vi "Test_uart.vi"() -> ()   [LabVIEW 2025]
uses:
  <vilib>/Instr/_visa.llb/VISA Configure Serial Port (Instr).vi
panel:
  in  "Stop Button":bool
  out "Waveform Chart":cluster{"Número":sgl, "Número":sgl}(graph)
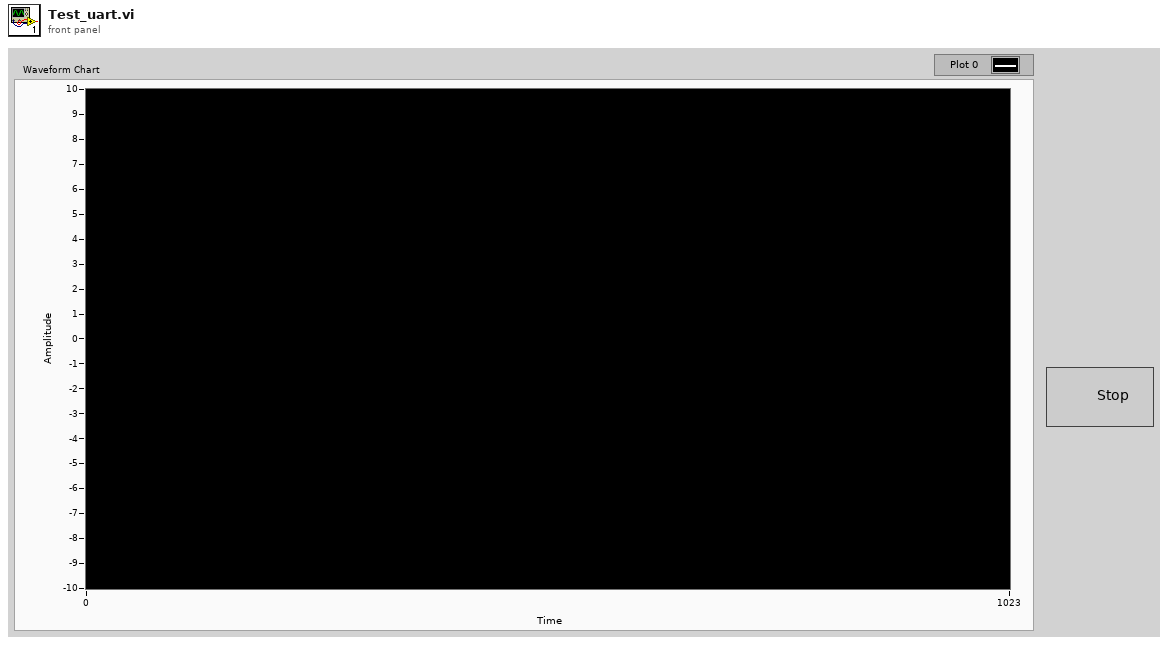
[diagram p1: front panel]
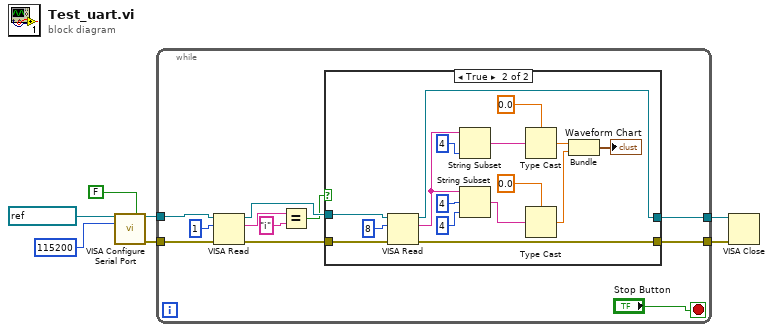
[diagram p0: block diagram]
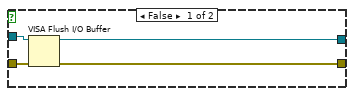
[diagram p2: hidden frame]
diagram:
  n1 = call-poly "VISA Configure Serial Port"("VISA resource name"=refnum<visa-resource-name> "COM14", "Enable Termination\nChar (T)"=FALSE ("Enable Termination\nChar (T)"), "baud rate (9600)"=u32 115200) -> ("VISA resource name out"=w2:refnum<visa-resource-name>, "error out"=w1:errorcluster)  [unwired: 11 in]
  n2 = while {
    tunnel: w2 -> [w14]
    tunnel: w1 -> [w13]
    tunnel: [w18] -> w7
    tunnel: [w17] -> w6
    stop <- "Stop Button" stop-if-true
    n3 = VISA Read(VISA resource name=w14, byte count=u32 1, error in (no error)=w13) -> (VISA resource name out=w12:refnum<visa-resource-name>, read buffer=w10:string, error out=w11:errorcluster)  [unwired: 1 out]
    n4 = Equal?(x=w10, y="i") -> (x = y?=w8:bool)
    n5 = case shown="True" w8 {
      tunnel: [w22 w38] -> w18
      tunnel: [w21 w37] -> w17
      tunnel: w12 -> [w20 w34]
      tunnel: w11 -> [w19 w33]
      frame False {
        n6 = VISA Flush I/O Buffer(VISA resource name=w20, error in (no error)=w19) -> (VISA resource name out=w22:refnum<visa-resource-name>, error out=w21:errorcluster)  [unwired: 1 in]
      }
      frame True {
        n7 = VISA Read(VISA resource name=w34, byte count=u32 8, error in (no error)=w33) -> (VISA resource name out=w38:refnum<visa-resource-name>, read buffer=w29:string, error out=w37:errorcluster)  [unwired: 1 out]
        n8 = String Subset(string=w29, length (rest)=4 ("length (rest)")) -> (substring=w31:string)  [unwired: 1 in]
        n9 = String Subset(string=w29, offset (0)=4, length (rest)=4 ("length (rest)")) -> (substring=w23:string)
        n10 = Type Cast(type=sgl 0.0 ("Número"), x=w31) -> (*(type *) &x=w27:sgl)
        n11 = Type Cast(type=sgl 0.0 ("Número"), x=w23) -> (*(type *) &x=w24:sgl)
        n12 = Bundle("Número"=w27, "Número"=w24) -> (→"Waveform Chart":cluster{"Número":sgl, "Número":sgl})  [unwired: 1 in]
      }
    }
  }
  n13 = VISA Close(VISA resource name=w7, error in (no error)=w6) -> ()  [unwired: 1 out]
